vi "Tree Control.vi"() -> ()   [LabVIEW 2019, in "Tree Map.lvlib"]
doc: "<b>Author:</b> Piotr Kruczkowski <PrimaryKey>\n<b>License:</b> NewBSD\n\nCopyright (c) 2019, National Instruments\nAll rights reserved.\n\nRedistribution and use in source and binary forms, with or without\nmodification, are permitted provided that the following conditions are met:\n1. Redistributions of source code must retain the above copyright\n notice, this list of conditions and the following disclaimer.\n2. Redistributions in binary form must reproduce the above copyright\n notice, this list of conditions and the following disclaimer in the\n documentation and/or other materials provided with the distribution.\n3. Neither the name of National Instruments nor the\n names of its contributors may be used to endorse or promote products\n derived from this software without specific prior written permission.\n\nTHIS SOFTWARE IS PROVIDED BY National Instruments ''AS IS'' AND ANY\nEXPRESS OR IMPLIED WARRANTIES, INCLUDING, BUT NOT LIMITED TO, THE IMPLIED\nWARRANTIES OF MERCHANTABILITY AND FITNESS FOR A PARTICULAR PURPOSE ARE\nDISCLAIMED. IN NO EVENT SHALL National Instruments BE LIABLE FOR ANY\nDIRECT, INDIRECT, INCIDENTAL, SPECIAL, EXEMPLARY, OR CONSEQUENTIAL DAMAGES\n(INCLUDING, BUT NOT LIMITED TO, PROCUREMENT OF SUBSTITUTE GOODS OR SERVICES;\nLOSS OF USE, DATA, OR PROFITS; OR BUSINESS INTERRUPTION) HOWEVER CAUSED AND\nON ANY THEORY OF LIABILITY, WHETHER IN CONTRACT, STRICT LIABILITY, OR TORT\n(INCLUDING NEGLIGENCE OR OTHERWISE) ARISING IN ANY WAY OUT OF THE USE OF THIS\nSOFTWARE, EVEN IF ADVISED OF THE POSSIBILITY OF SUCH DAMAGE."
uses:
  Tree Map.lvlib
  API/List Roots.vi
  Utility/Into Tree Control Items.vi
panel:
  out "Node Data":T1={"Child Paths Set"={}, "Name"="MySubNode", "Data"="0.68", "Attributes"={}}
  out "Node Path":string="\\Root\\MyNode\\MySubNode"
  in  "Tree Control - Click on the elements":string(tree)="\\Root\\MyNode\\MySubNode"
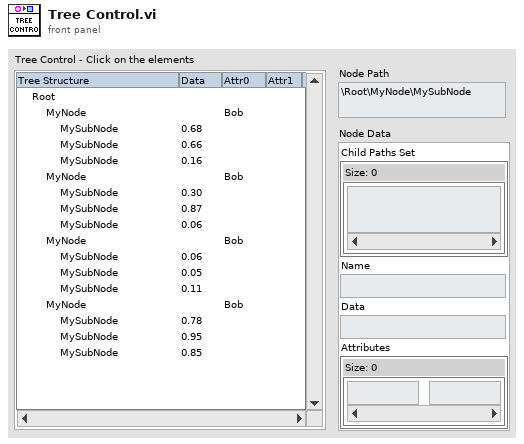
[diagram p1: front panel]
types:
  T1 = cluster{"Child Paths Set":set{string}, "Name":string, "Data":string, "Attributes":map{string, string}}
  T2 = typedef "Tree Map.lvlib/Tree Map Data.ctl" = map{string, cluster{"Child Paths Set":set{string}, "Name":string, "Data":string, "Attributes":map{string, string}}}
  T3 = cluster{"Left Cell String":string, "Child Text":string[], "Child Tag":string, "Item Indent":i32, "Child Only?":bool, "Glyph Index":i32}[]
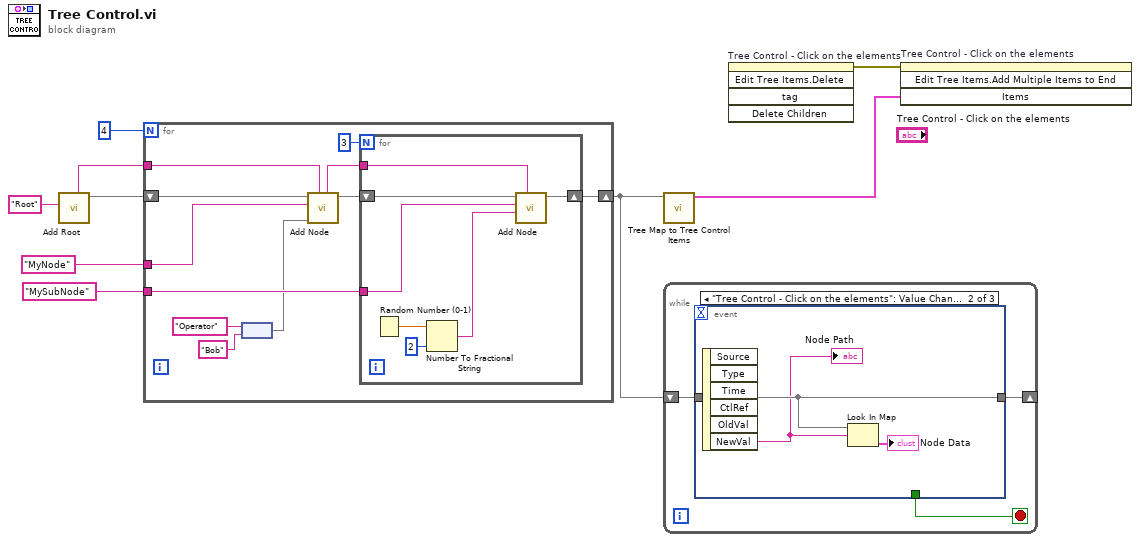
[diagram p0: block diagram]
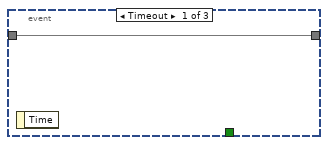
[diagram p2: hidden frame]
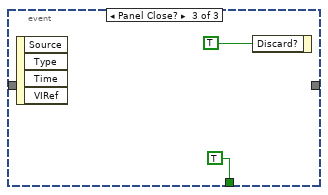
[diagram p3: hidden frame]
diagram:
  n1 = call "Add Root.vi"("New Root Name"="Root") -> ("Tree Map Out"=w9:T2, "Root Path"=w8:string)  [unwired: 9 in]
  n2 = for {
    N: 4 -> [_]
    tunnel: w8 -> [w19]
    tunnel: "MyNode" ("New Node Name") -> [w18]
    shift-right: [w17] -> w1
    shift-left: w9 -> [w20]
    tunnel: "MySubNode" ("New Node Name") -> [w14]
    n3 = node("Operator" ("key"), "Bob" ("key")) -> (w10:map{string, string})
    n4 = call "Add Node.vi"("Parent Path"=w19, "Attributes"=w10, "New Node Name"=w18, "Tree Map In"=w20) -> ("Tree Map Out"=w16:T2, "New Node Path"=w15:string)  [unwired: 5 in, 1 out]
    n5 = for {
      N: 3 -> [_]
      shift-right: [w26] -> w17
      shift-left: w16 -> [w27]
      tunnel: w15 -> [w25]
      tunnel: w14 -> [w24]
      n6 = Random Number (0-1)() -> (number: 0 to 1=w23:dbl)
      n7 = Number To Fractional String(number=w23, precision (6)=i16 2) -> (F-format string=w21:string)  [unwired: 2 in]
      n8 = call "Add Node.vi"("Parent Path"=w25, "Data"=w21, "New Node Name"=w24, "Tree Map In"=w27) -> ("Tree Map Out"=w26:T2)  [unwired: 5 in, 2 out]
    }
  }
  n9 = call "Tree Map to Tree Control Items.vi"("Tree Map In"=w1) -> ("Tree Control Items"=w2:T3)  [unwired: 10 in]
  n10 = while {
    shift-right: [w30] -> _
    shift-left: w1 -> [w29]
    stop <- w28 stop-if-true
    n11 = event shown="[1] \"Tree Control - Click on the elements\": Value Change" {
      selector: _ -> [_ _ _]
      dyn-events: _ -> [_ _ _]
      timeout: _ -> [_ _ _]
      tunnel: [w31 w34 _] -> w30
      tunnel: w29 -> [w31 w34 _]
      tunnel: [_ _ TRUE ("Discard?")] -> w28
      event Timeout {
        n12 = event-data() -> ()  [unwired: 1 in, 1 out]
      }
      event "Tree Control - Click on the elements": Value Change {
        n13 = event-data() -> ("NewVal"=w32:string)  [unwired: 1 in, 5 out]
        "Node Path" <- w32
        n14 = Look In Map(map=w34, key=w32) -> (value=→"Node Data":T1)  [unwired: 1 in, 1 out]
      }
      event Panel Close? {
        n15 = event-data() -> ()  [unwired: 1 in, 4 out]
        n16 = event-data("Discard?"=TRUE) -> ()  [unwired: 1 in, 1 out]
      }
    }
  }
  n17 = invoke on="Tree Control - Click on the elements" class="Tree (strict)" method="Edit Tree Items.Delete"() -> (error out=w6:errorcluster)  [unwired: 5 in, 4 out]
  n18 = invoke on="Tree Control - Click on the elements" class="Tree (strict)" method="Edit Tree Items.Add Multiple Items to End"(error in=w6, "Items"=w2) -> ()  [unwired: 2 in, 4 out]
